vi "Z Aux Get Modbus In.vi"(7 "pValueList":string, 8 "error in (no error)":errorcluster caption="错误输入（无错误）", 9 "ionumend":i32, 10 "ionumfirst":i32, 11 "handle":u32) -> (0 "error out":errorcluster caption="错误输出", 2 "function return":i32, 3 "handle out":u32, 5 "pValueList out":string)   [LabVIEW 2015, in "zauxdll.lvlib"]
doc: "int32 __stdcall ZAux_GetModbusIn(ZMC_HANDLE handle, int ionumfirst, int ionumend, uint8 pValueList[]);"
uses:
  zauxdll.lvlib
  zauxdll.dll
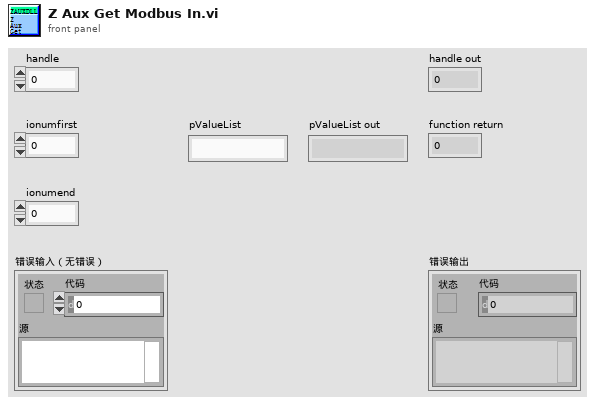
[diagram p1: front panel]
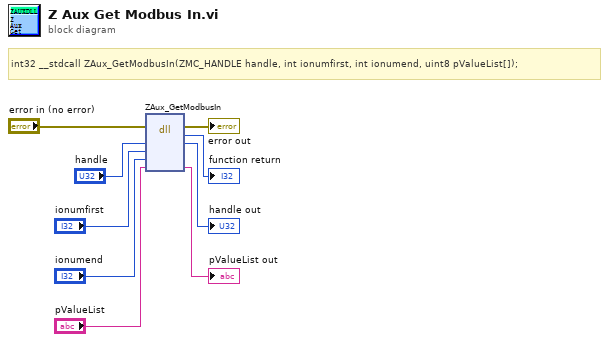
[diagram p0: block diagram]
diagram:
  # "int32 __stdcall ZAux_GetModbusIn(ZMC_HANDLE handle, int ionumfirst, int ionumend, uint8 pValueList[]);"
  n1 = dll-call lib="D:/vicomm case/cub/0717/15/Main Folder/Radar - 2015 32bit_autoqueue_angle_0319/zauxdll-2014/zauxdll.dll" fn="ZAux_GetModbusIn"(error in="error in (no error)", "handle"="handle", "ionumfirst"="ionumfirst", "ionumend"="ionumend", "pValueList"="pValueList") -> (error out=→"error out":errorcluster, "return type"=→"function return":i32, "handle"=→"handle out":u32, "pValueList"=→"pValueList out":string)  [unwired: 4 in, 1 out]
